vi "GetVisionHub.vi"() -> (13 "Vision Timestamp (ms)":u32, 14 "Vision Horizontal Angle to Target (deg) [t-?]":dbl, 15 "Vision Vertical Angle to Target (deg) [t-?]":dbl, 16 "Vision Target Valid [t-?]":bool)   [LabVIEW 2020]
doc: "Reads the raw data from the LimeLight used for targeting the LimeLight. Performs some minor transformations and conducts intial validity checks."
uses:
  2d64956e-cf35-4d84-838e-e30eff74bf58.vi
  <vilib>/Rock Robotics/Network Tables/NT Read Number.vi
  driverdata.vi
  sensordata.vi
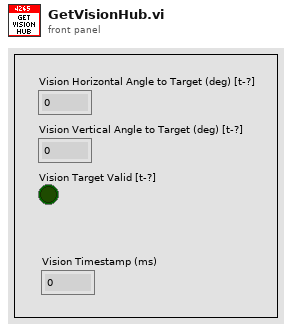
[diagram p1: front panel]
types:
  T1 = enum16{"Boot Up", "Camera Override", "HUB Targeting", "CARGO Tracking"}
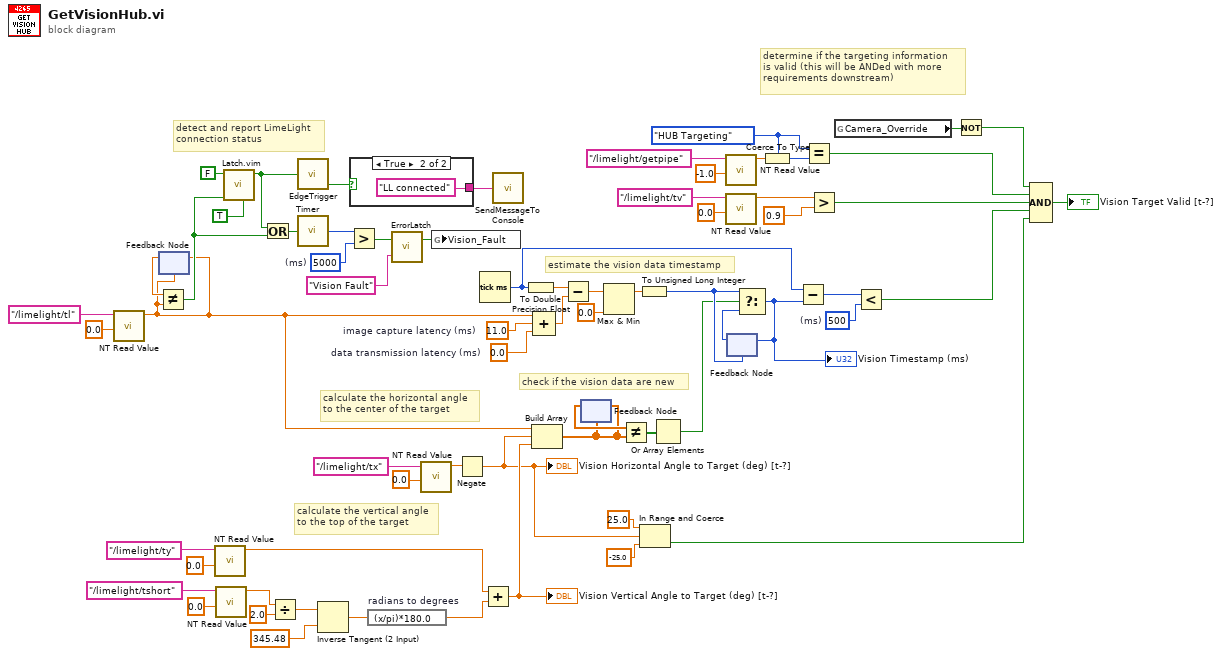
[diagram p0: block diagram]
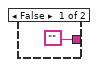
[diagram p2: hidden frame]
diagram:
  w4 = 0.0  # data transmission latency (ms)
  w17 = u32 5000  # (ms)
  w23 = u32 500  # (ms)
  w39 = 11.0  # image capture latency (ms)
  w53 = T1."HUB Targeting" ("x")
  # "detect and report LimeLight\nconnection status"
  # "calculate the horizontal angle\nto the center of the target"
  # "determine if the targeting information\nis valid (this will be ANDed with more\nrequirements downstream)"
  # "calculate the vertical angle\nto the top of the target"
  # "estimate the vision data timestamp"
  # "check if the vision data are new"
  n1 = call-poly <vilib>:"NT Read Value.vi"("Default Value"=0.0, "Name"="/limelight/tl") -> ("Numeric"=w1:dbl)  [unwired: 8 in, 1 out]
  n2 = feedback-in #1(w1) -> ()
  n3 = feedback #1(w1) -> (w20:dbl)
  n4 = Not Equal?(x=w20, y=w1) -> (x != y?=w14:bool)
  n5 = call-poly <vilib>:"NT Read Value.vi"("Default Value"=0.0, "Name"="/limelight/ty") -> ("Numeric"=w43:dbl)  [unwired: 8 in, 1 out]
  n6 = call-poly <vilib>:"NT Read Value.vi"("Default Value"=0.0, "Name"="/limelight/tshort") -> ("Numeric"=w44:dbl)  [unwired: 8 in, 1 out]
  n7 = call "Latch.vim"("Default Value"=TRUE, "Latch Signal"=w14, "Latch Value"=FALSE) -> ("Latched"=w11:bool)  [unwired: 8 in]
  n8 = Or(x=w11, y=w14) -> (x .or. y?=w16:bool)
  n9 = Divide(x=w44, y=2.0) -> (x/y=w47:dbl)
  n10 = call "EdgeTrigger.vi"("Input Signal"=w11) -> ("Falling Edge Trigger"=w9:bool)  [unwired: 2 out]
  n11 = call "Timer.vi"("Reset Timer"=w16) -> ("Time (ms)"=w18:u32)
  n12 = Inverse Tangent (2 Input)(1:345.48 ("x"), 2:w47) -> (0:w46:dbl)
  n13 = Greater?(x=w18, y=w17) -> (0:w19:bool)
  n14 = case shown="True" w9 {
    tunnel: ["" "LL connected" ("Message")] -> w10
    frame False {
    }
    frame True {
    }
  }
  n15 = expression code="(x/pi)*180.0" "radians to degrees"(w46) -> (w45:dbl)
  n16 = call "ErrorLatch.vi"("Error Message"="Vision Fault", "Trigger"=w19) -> ("Latched"=w12:bool)  [unwired: 1 in]
  n17 = call-poly <vilib>:"NT Read Value.vi"("Default Value"=0.0, "Name"="/limelight/tx") -> ("Numeric"=w59:dbl)  [unwired: 8 in, 1 out]
  n18 = global write "sensordata.vi" "Vision_Fault"(w12) -> ()
  n19 = Negate(x=w59) -> (-x=w2:dbl)
  "Vision Horizontal Angle to Target (deg) [t-?]" <- w2
  n20 = Tick Count (ms)() -> (millisecond timer value=w26:u32)
  n21 = Add(x=w43, y=w45) -> (x+y=w31:dbl)
  "Vision Vertical Angle to Target (deg) [t-?]" <- w31
  n22 = call "SendMessageToConsole.vi"("Message String"=w10) -> ()  [unwired: 1 in]
  n23 = To Double Precision Float(number=w26) -> (double precision float=w37:dbl)
  n24 = Build Array(w1, w2, w31) -> (w30:dbl[])
  n25 = Compound Arithmetic op=ADD(w1, w39, w4) -> (w38:dbl)
  n26 = Subtract(x=w37, y=w38) -> (x-y=w36:dbl)
  n27 = feedback-in #2(w30) -> ()
  n28 = feedback #2(w30) -> (w32:dbl[])
  n29 = Max & Min(x=w36, y=0.0) -> (max(x,y)=w34:dbl)  [unwired: 1 out]
  n30 = Not Equal?(x=w32, y=w30) -> (x != y?=w29:bool[])
  n31 = To Unsigned Long Integer(number=w34) -> (unsigned 32bit integer=w33:u32)
  n32 = In Range and Coerce(upper limit=25.0, x=w2, lower limit=-25.0) -> (In Range?=w5:bool)  [unwired: 1 out]
  n33 = Or Array Elements(Boolean array=w29) -> (logical OR=w28:bool)
  n34 = call-poly <vilib>:"NT Read Value.vi"("Default Value"=-1.0, "Name"="/limelight/getpipe") -> ("Numeric"=w56:dbl)  [unwired: 8 in, 1 out]
  n35 = call-poly <vilib>:"NT Read Value.vi"("Default Value"=0.0, "Name"="/limelight/tv") -> ("Numeric"=w63:dbl)  [unwired: 8 in, 1 out]
  n36 = feedback #3(w33) -> (w40:u32)
  n37 = Select(t=w33, s=w28, f=w40) -> (s? t:f=w27:u32)
  "Vision Timestamp (ms)" <- w27
  n38 = feedback-in #3(w27) -> ()
  n39 = Coerce To Type(0:w56, 1:w53) -> (2:w55:T1)
  n40 = Subtract(x=w26, y=w27) -> (x-y=w25:u32)
  n41 = Equal?(x=w53, y=w55) -> (x = y?=w54:bool)
  n42 = Greater?(x=w63, y=0.9) -> (0:w52:bool)
  n43 = global read "driverdata.vi" "Camera_Override"() -> (w22:bool)
  n44 = Less?(x=w25, y=w23) -> (x < y?=w24:bool)
  n45 = Not(x=w22) -> (.not. x?=w21:bool)
  n46 = Compound Arithmetic op=AND(w21, w54, w52, w24, w5) -> (→"Vision Target Valid [t-?]":bool)
